vi "JSON RPC Server.vi"() -> ()   [LabVIEW 2020]
uses:
  Lib/JSON-RPC/Classes/Server/JSONRPC Server.lvclass
  Controller/Controller.lvclass
  Lib/JSON-RPC/Classes/Server/Add Response (Result from Request).vi
  Lib/JSON-RPC/Classes/Server/Add Response (Server Error from Request).vi
  Lib/JSON-RPC/Classes/Server/Send Request (Sync).vi
  Lib/JSON-RPC/Classes/Server/Add Response (Internal Error from Request).vi
panel:
  out "header":string
  out "request":string
  out "response":string
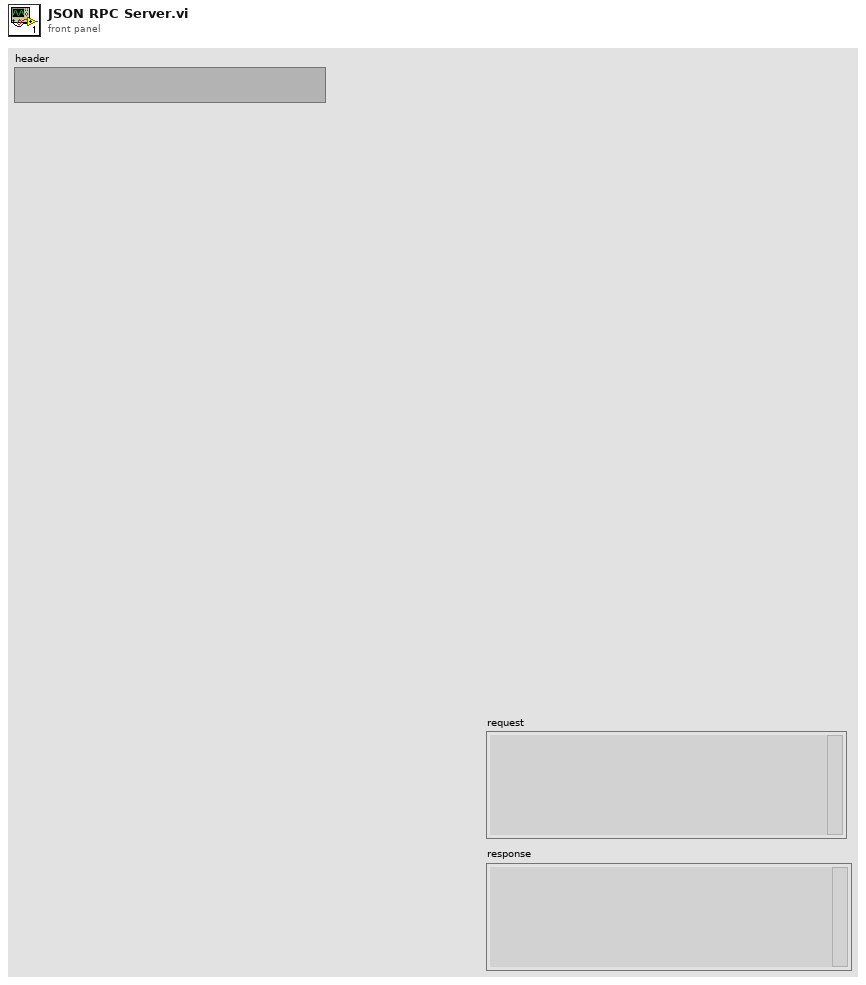
[diagram p1: front panel]
types:
  T1 = enum16{"Standard", "Buffered", "CRLF", "Immediate"}
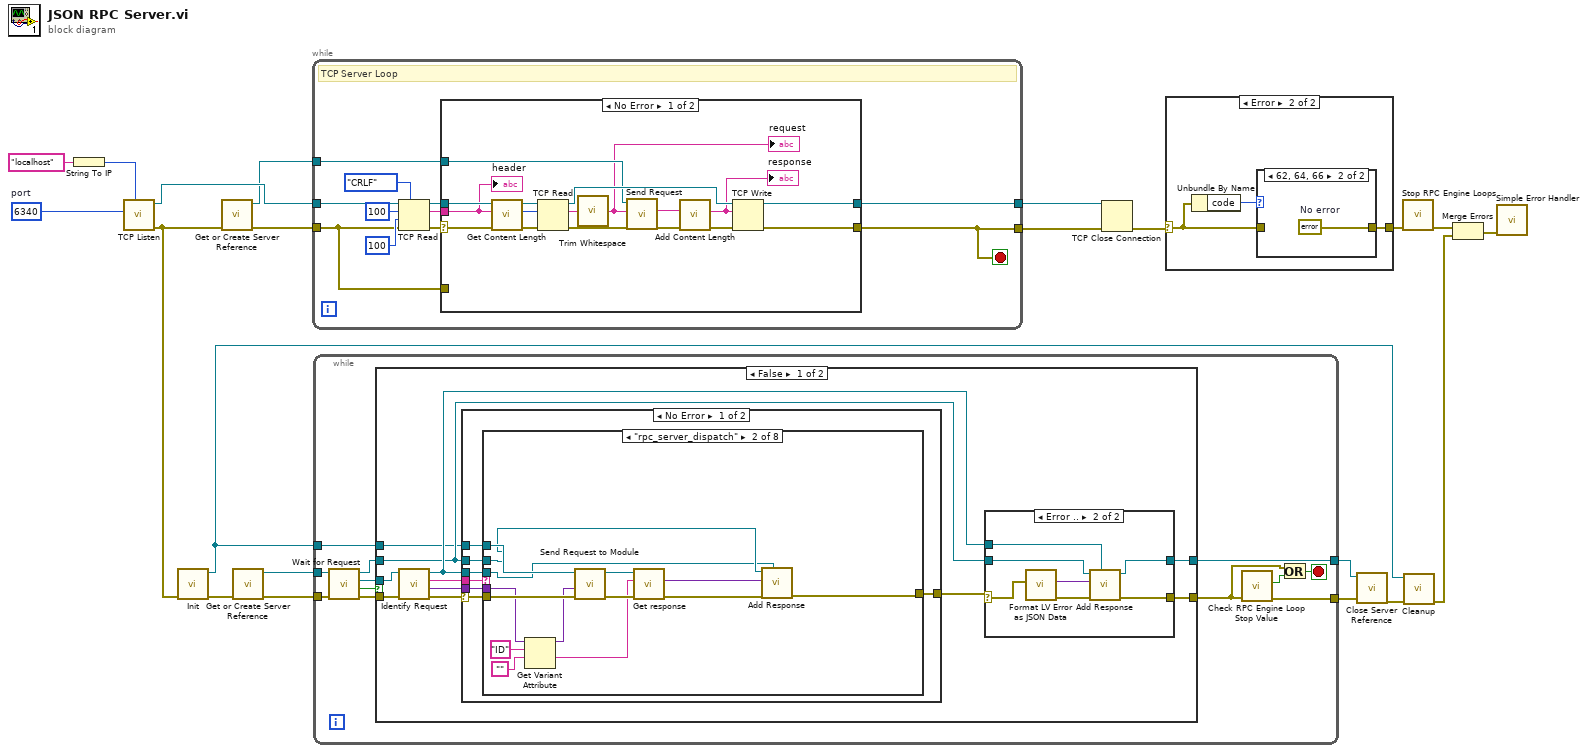
[diagram p0: block diagram]
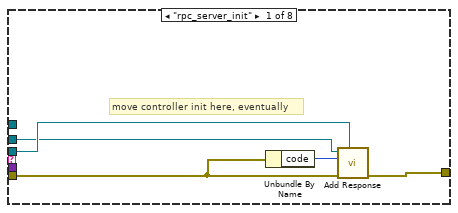
[diagram p3: hidden frame]
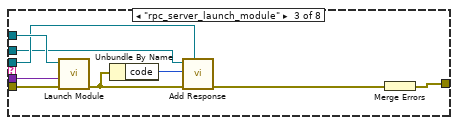
[diagram p4: hidden frame]
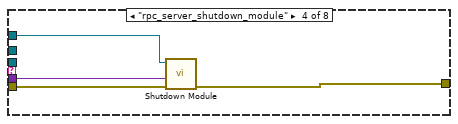
[diagram p5: hidden frame]
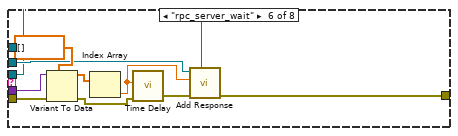
[diagram p7: hidden frame]
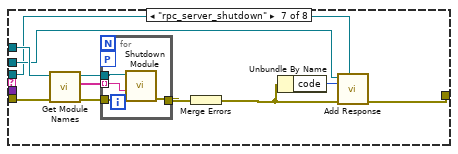
[diagram p8: hidden frame]
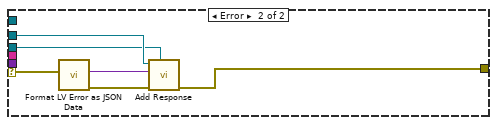
[diagram p10: hidden frame]
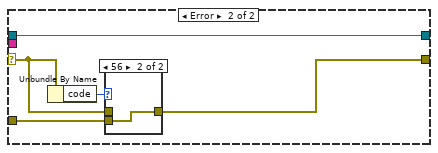
[diagram p14: hidden frame]
diagram:
  w19 = u16 6340  # port
  n1 = String To IP(1:"localhost" ("name")) -> (0:w18:u32)
  n2 = call <vilib>:"TCP Listen.vi"("net address"=w18, "port"=w19) -> ("error out"=w6:errorcluster, "connection ID"=w15:refnum<k5>)  [unwired: 5 in, 3 out]
  n3 = call "Init.vi"("error in (no error)"=w6) -> ("error out"=w1:errorcluster, "Controller out"=w2:refnum<class "Controller.lvclass">)  [unwired: 9 in]
  n4 = call "Get or Create Server Reference.vi"("error in (no error)"=w6) -> ("error out"=w14:errorcluster, "Server Out"=w13:refnum<class "JSONRPC Server.lvclass">)  [unwired: 9 in]
  n5 = call "Get or Create Server Reference.vi"("error in (no error)"=w1) -> ("error out"=w11:errorcluster, "Server Out"=w3:refnum<class "JSONRPC Server.lvclass">)  [unwired: 9 in]
  n6 = while {
    tunnel: [w22] -> w20
    tunnel: [w29] -> w21
    tunnel: w15 -> [w25]
    tunnel: w14 -> [w26]
    tunnel: w13 -> [w23]
    stop <- w22 stop-if-true
    # "TCP Server Loop"
    n7 = TCP Read(connection ID=w25, bytes to read=100, error in (no error)=w26, 7:T1."CRLF" ("mode (standard)"), 9:100 ("timeout ms (25000)")) -> (connection ID out=w30:refnum<k5>, data out=w24:string, error out=w28:errorcluster)
    n8 = case shown="No Error" w28 {
      selector: w28 -> [w48 w52]
      tunnel: [w42 w50] -> w22
      tunnel: w26 -> [_ w51]
      tunnel: [w43 w49] -> w29
      tunnel: w30 -> [w46 w49]
      tunnel: w24 -> [w45 _]
      tunnel: w23 -> [w39 _]
      frame No Error {
        n9 = call "Get Content Length.vi"("error in (no error)"=w48, "header"=w45) -> ("error out"=w47:errorcluster, "content length"=w44:i32)  [unwired: 8 in]
        n10 = TCP Read(connection ID=w46, bytes to read=w44, error in (no error)=w47) -> (connection ID out=w41:refnum<k5>, data out=w34:string, error out=w40:errorcluster)  [unwired: 2 out]
        n11 = call <vilib>:"Trim Whitespace.vi"("string"=w34) -> ("trimmed string"=w33:string)  [unwired: 1 in]
        "request" <- w33
        n12 = call-poly "Send Request.vi"("error in (no error)"=w40, "JSON Request String"=w33, "JSONRPC Server in"=w39) -> ("error out"=w38:errorcluster, "JSON Response String"=w35:string)  [unwired: 6 in, 1 out]
        n13 = call "Add Content Length.vi"("error in (no error)"=w38, "JSON Response String in"=w35) -> ("error out"=w37:errorcluster, "JSON Response String out"=w36:string)  [unwired: 8 in]
        "response" <- w36
        n14 = TCP Write(connection ID=w41, data in=w36, error in (no error)=w37) -> (connection ID out=w43:refnum<k5>, error out=w42:errorcluster)  [unwired: 1 in, 1 out]
        "header" <- w45
      }
      frame Error {
        n15 = Unbundle By Name(w52) -> ("code"=w53:i32)
        n16 = case shown="56" w53 {
          tunnel: w52 -> [w54 _]
          tunnel: w51 -> [_ w55]
          tunnel: [w54 w55] -> w50
          frame Default {
          }
          frame 56 {
          }
        }
      }
    }
  }
  n17 = while {
    tunnel: w11 -> [w67]
    tunnel: w3 -> [w66]
    tunnel: [w61] -> w10
    tunnel: [w60] -> w9
    tunnel: w2 -> [w56]
    stop <- w57 stop-if-true
    n18 = call "Wait for Request.vi"("error in (no error)"=w67, "Server in"=w66) -> ("error out"=w65:errorcluster, "timed out?"=w62:bool, "Request"=w64:refnum<class "Request.lvclass">, "Server out"=w63:refnum<class "JSONRPC Server.lvclass">)  [unwired: 6 in]
    n19 = case shown="False" w62 {
      tunnel: w65 -> [w71 w161]
      tunnel: w64 -> [w78 _]
      tunnel: w63 -> [w69 w160]
      tunnel: [w74 w161] -> w58
      tunnel: [w73 w160] -> w60
      tunnel: w56 -> [w68 _]
      frame False {
        n20 = call "Identify Request.vi"("error in (no error)"=w71, "Request in"=w78) -> ("error out"=w72:errorcluster, "params"=w77:variant, "method"=w70:string, "Request out"=w75:refnum<class "Request.lvclass">)  [unwired: 5 in, 1 out]
        n21 = case shown="No Error" w72 {
          selector: w72 -> [w92 w159]
          tunnel: w77 -> [w89 _]
          tunnel: w69 -> [w94 w157]
          tunnel: w75 -> [w93 w156]
          tunnel: [w91 w154] -> w76
          tunnel: w70 -> [w90 _]
          tunnel: w68 -> [w88 _]
          frame No Error {
            n22 = case shown="\"rpc_server_dispatch\"" w90 {
              tunnel: w94 -> [w97 w109 w116 _ _ w131 w140 _]
              tunnel: w93 -> [w98 w102 w117 _ _ w129 w138 _]
              tunnel: w92 -> [w96 w113 w122 w126 w127 w137 w143 w153]
              tunnel: [w99 w110 w121 w125 w127 w128 w139 w153] -> w91
              tunnel: w89 -> [_ w105 w119 w123 _ w136 _ _]
              tunnel: w88 -> [_ w112 w120 w124 _ _ w144 _]
              frame "rpc_server_init" {
                # "move controller init here, eventually"
                n23 = Unbundle By Name(w96) -> ("code"=w95:i32)
                n24 = call-poly "Add Response.vi"("Request"=w98, "error in (no error)"=w96, "JSON Value in"=w95, "Server in"=w97) -> ("error out"=w99:errorcluster)  [unwired: 5 in, 2 out]
              }
              frame "rpc_server_dispatch" {
                n25 = Get Variant Attribute(Variant=w105, name="ID", default value (empty Variant)="") -> (duplicate Variant=w104:variant, value=w103:string)  [unwired: 1 in, 2 out]
                n26 = call "Send Request to Module.vi"("error in (no error)"=w113, 9:w104, "Controller in"=w112) -> ("error out"=w108:errorcluster, "Controller out"=w111:refnum<class "Controller.lvclass">)  [unwired: 6 in, 1 out]
                n27 = call "Get response.vi"("error in"=w108, "Request"=w103, "Controller in"=w111) -> ("error out"=w101:errorcluster, "Response"=w100:variant)  [unwired: 5 in, 2 out]
                n28 = call-poly "Add Response.vi"("Request"=w102, "error in (no error)"=w101, "JSON Value in"=w100, "Server in"=w109) -> ("error out"=w110:errorcluster)  [unwired: 5 in, 2 out]
              }
              frame "rpc_server_launch_module" {
                n29 = call "Launch Module.vi"("error in (no error)"=w122, "params"=w119, "Controller in"=w120) -> ("error out"=w115:errorcluster)  [unwired: 7 in, 1 out]
                n30 = Unbundle By Name(w115) -> ("code"=w114:i32)
                n31 = call-poly "Add Response.vi"("Request"=w117, "error in (no error)"=w115, "JSON Value in"=w114, "Server in"=w116) -> ("error out"=w118:errorcluster)  [unwired: 5 in, 2 out]
                n32 = Merge Errors(w118) -> (w121:errorcluster)
              }
              frame "rpc_server_shutdown_module" {
                n33 = call "Shutdown Module.vi"("error in (no error)"=w126, "params"=w123, "Controller in"=w124) -> ("error out"=w125:errorcluster)  [unwired: 7 in, 1 out]
              }
              frame "rpc_server_broadcast" {
              }
              frame "rpc_server_wait" {
                n34 = Variant To Data(error in=w137, type=dbl[] [], Variant=w136) -> (data=w134:dbl[], error out=w133:errorcluster)
                n35 = Index Array(array=w134) -> (element=w130:dbl)  [unwired: 1 in]
                n36 = call "Time Delay"("error in (no error)"=w133, "Delay Time (s)"=w130) -> ("error out"=w132:errorcluster)  [unwired: 9 in]
                n37 = call-poly "Add Response.vi"("Request"=w129, "error in (no error)"=w132, "JSON Value in"=w130, "Server in"=w131) -> ("error out"=w128:errorcluster)  [unwired: 5 in, 2 out]
              }
              frame "rpc_server_shutdown" {
                n38 = call "Get Module Names.vi"("error in (no error)"=w143, "Controller in"=w144) -> ("error out"=w147:errorcluster, "Names"=w148:string[], "Controller out"=w145:refnum<class "Controller.lvclass">)  [unwired: 7 in]
                n39 = for {
                  tunnel: w145 -> [w152]
                  tunnel: w148 -> [w149] mode=indexing
                  tunnel: w147 -> [w151]
                  tunnel: [w150] -> _ mode=indexing
                  tunnel: [w150] -> w146
                  workers-P: _ -> [_]
                  n40 = call "Shutdown Module.vi"("error in (no error)"=w151, "params"=w149, "Controller in"=w152) -> ("error out"=w150:errorcluster)  [unwired: 7 in, 1 out]
                }
                n41 = Merge Errors(w146) -> (w142:errorcluster)
                n42 = Unbundle By Name(w142) -> ("code"=w141:i32)
                n43 = call-poly "Add Response.vi"("Request"=w138, "error in (no error)"=w142, "JSON Value in"=w141, "Server in"=w140) -> ("error out"=w139:errorcluster)  [unwired: 5 in, 2 out]
              }
              frame Default {
              }
            }
          }
          frame Error {
            n44 = call "Format LV Error as JSON Data.vi"("error in"=w159) -> ("error out"=w158:errorcluster, "Error Value out"=w155:variant)  [unwired: 9 in]
            n45 = call-poly "Add Response.vi"("Request"=w156, "error in (no error)"=w158, "data"=w155, "Server in"=w157) -> ("error out"=w154:errorcluster)  [unwired: 5 in, 2 out]
          }
        }
        n46 = case shown="Error .." w76 {
          selector: w76 -> [w80 w85]
          tunnel: [w80 w84] -> w74
          tunnel: w69 -> [w79 w82]
          tunnel: [w79 w83] -> w73
          tunnel: w75 -> [_ w81]
          frame No Error {
          }
          frame Error {
            n47 = call "Format LV Error as JSON Data.vi"("error in"=w85) -> ("error out"=w87:errorcluster, "Error Value out"=w86:variant)  [unwired: 9 in]
            n48 = call-poly "Add Response.vi"("Request"=w81, "error in (no error)"=w87, "data"=w86, "Server in"=w82) -> ("error out"=w84:errorcluster, "Server out"=w83:refnum<class "JSONRPC Server.lvclass">)  [unwired: 5 in, 1 out]
          }
        }
      }
      frame True {
      }
    }
    n49 = call "Check RPC Engine Loop Stop Value.vi"("error in (no error)"=w58) -> ("error out"=w61:errorcluster, "stopped?"=w59:bool)  [unwired: 9 in]
    n50 = Or(x=w58, y=w59) -> (x .or. y?=w57:bool)
  }
  n51 = TCP Close Connection(connection ID=w21, error in (no error)=w20) -> (error out=w17:errorcluster)  [unwired: 2 out]
  n52 = case shown="Error" w17 {
    selector: w17 -> [w162 w164]
    tunnel: [w162 w163] -> w12
    frame No Error {
    }
    frame Error {
      n53 = Unbundle By Name(w164) -> ("code"=w165:i32)
      n54 = case shown="62, 64, 66" w165 {
        tunnel: w164 -> [w166 _]
        tunnel: [w166 w167] -> w163
        frame Default {
        }
        frame 62, 64, 66 {
          w167 = errorcluster {"status"=FALSE, "code"=0, "source"=""}  # No error
        }
      }
    }
  }
  n55 = call "Close Server Reference.vi"("error in (no error)"=w10, "Server in"=w9) -> ("error out"=w5:errorcluster)  [unwired: 9 in]
  n56 = call "Stop RPC Engine Loops.vi"("error in (no error)"=w12) -> ("error out"=w8:errorcluster)  [unwired: 10 in]
  n57 = call "Cleanup.vi"("error in (no error)"=w5, "Controller in"=w2) -> ("error out"=w4:errorcluster)  [unwired: 9 in]
  n58 = Merge Errors(w8, w4) -> (w7:errorcluster)
  n59 = call <vilib>:"Simple Error Handler.vi"("error in (no error)"=w7) -> ()  [unwired: 1 in, 8 out]
